vi "Calculator.vi"() -> ()   [LabVIEW 2021]
panel:
  in  "Calculator":T1
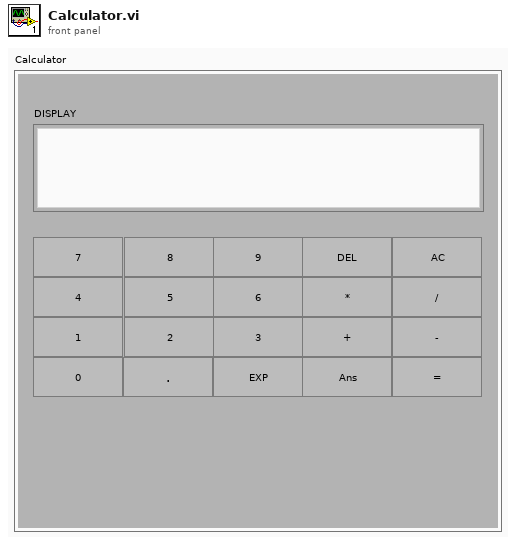
[diagram p1: front panel]
types:
  T1 = cluster{"1":bool, "2":bool, "3":bool, "4":bool, "5":bool, "6":bool, "7":bool, "8":bool, "9":bool, "0":bool, "3 2":bool, "3 3":bool, "6 2":bool, "9 2":bool, "3 4":bool, "6 3":bool, "9 3":bool, "3 5":bool, "6 4":bool, "9 4":bool, "DISPLAY":string}
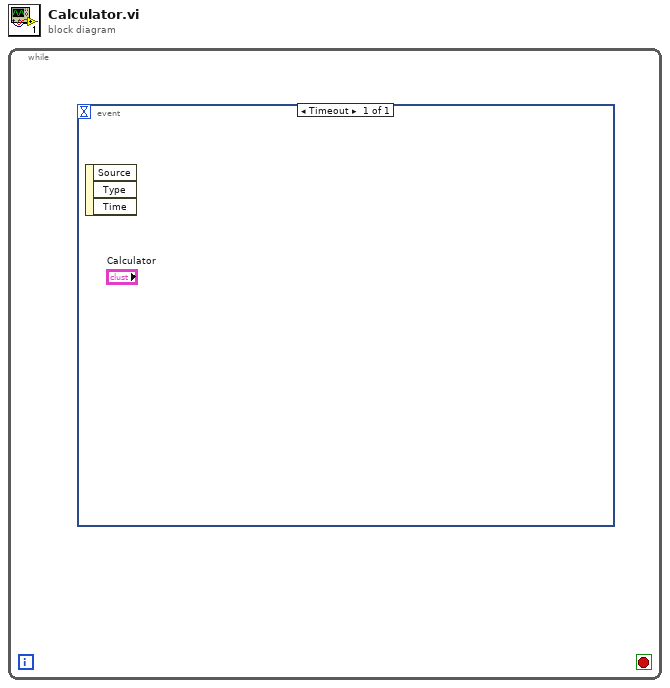
[diagram p0: block diagram]
diagram:
  n1 = while {
    stop <- _ stop-if-true
    n2 = event shown="[0] Timeout" {
      selector: _ -> [_]
      dyn-events: _ -> [_]
      timeout: _ -> [_]
      event Timeout {
        n3 = event-data() -> ()  [unwired: 1 in, 3 out]
      }
    }
  }
